vi "testArbNiTwoTone.vi"   [LabVIEW 2023]
uses:
  ArbNi.lvclass
  Data/arbWaveformType.ctl
  sweArb.lvlib
types:
  T1 = typedef "sweArb.lvlib/arbWaveformType.ctl" = enum16{"Sine", "Square", "Triangle", "DC", "Noise", "Arb"}
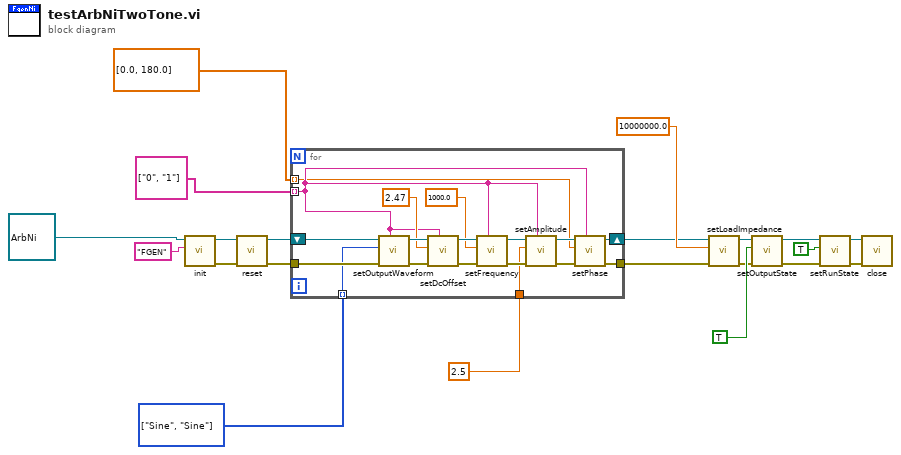
[diagram p0: block diagram]
diagram:
  w1 = T1[] [enum."Sine", enum."Sine"] items=["Sine", "Square", "Triangle", "DC", "Noise", "Arb"] ("Array")
  w9 = 10000000.0 items=["50 Ohm"=50.0, "High Z"=10000000.0] ("Load Impedance")
  n1 = call-dynamic "init.vi"("Resource"="FGEN", "FgenNiPxi in"=refnum<class "ArbNi.lvclass"> refnum) -> ("error out"=w20:errorcluster, "FgenNiPxi out"=w21:refnum<class "ArbNi.lvclass">)  [unwired: 8 in]
  n2 = call-dynamic "reset.vi"("error in (no error)"=w20, "FgenNiPxi in"=w21) -> ("error out"=w18:errorcluster, "FgenNiPxi out"=w19:refnum<class "ArbNi.lvclass">)  [unwired: 8 in]
  n3 = for {
    tunnel: w18 -> [w38]
    tunnel: [w30] -> w6
    tunnel: string[] ["0", "1"] ("Channel") -> [w26] mode=indexing
    tunnel: dbl[] [0.0, 180.0] ("Phase [°]") -> [w24] mode=indexing
    shift-right: [w31] -> w7
    shift-left: w19 -> [w39]
    tunnel: 2.5 ("Amplitude [Vpk]") -> [w23]
    tunnel: w1 -> [w22] mode=indexing
    n4 = call-dynamic "setOutputWaveform.vi"("Channel"=w26, "error in (no error)"=w38, "Type"=w22, "FgenNiPxi in"=w39) -> ("error out"=w36:errorcluster, "FgenNiPxi out"=w37:refnum<class "ArbNi.lvclass">)  [unwired: 6 in]
    n5 = call-dynamic "setDcOffset.vi"("Channel"=w26, "error in (no error)"=w36, "Offset [V]"=2.47, "FgenNiPxi in"=w37) -> ("error out"=w34:errorcluster, "FgenNiPxi out"=w35:refnum<class "ArbNi.lvclass">)  [unwired: 6 in]
    n6 = call-dynamic "setFrequency.vi"("Channel"=w26, "error in (no error)"=w34, "Frequency [Hz]"=1000.0, "FgenNiPxi in"=w35) -> ("error out"=w32:errorcluster, "FgenNiPxi out"=w33:refnum<class "ArbNi.lvclass">)  [unwired: 6 in]
    n7 = call-dynamic "setAmplitude.vi"("Channel"=w26, "error in (no error)"=w32, "Amplitude [Vpkpk]"=w23, "FgenNiPxi in"=w33) -> ("error out"=w25:errorcluster, "FgenNiPxi out"=w27:refnum<class "ArbNi.lvclass">)  [unwired: 6 in]
    n8 = call-dynamic "setPhase.vi"("Channel"=w26, "error in (no error)"=w25, "Phase [°]"=w24, "FgenNiPxi in"=w27) -> ("error out"=w30:errorcluster, "FgenNiPxi out"=w31:refnum<class "ArbNi.lvclass">)  [unwired: 6 in]
  }
  n9 = call-dynamic "setLoadImpedance.vi"("error in (no error)"=w6, "Load Impedance"=w9, "FgenNiPxi in"=w7) -> ("error out"=w5:errorcluster, "FgenNiPxi out"=w4:refnum<class "ArbNi.lvclass">)  [unwired: 7 in]
  n10 = call-dynamic "setOutputState.vi"("error in (no error)"=w5, "Output State"=TRUE, "FgenNiPxi in"=w4) -> ("error out"=w3:errorcluster, "FgenNiPxi out"=w17:refnum<class "ArbNi.lvclass">)  [unwired: 7 in]
  n11 = call-dynamic "setRunState.vi"("error in (no error)"=w3, "Runstate"=TRUE, "FgenNiPxi in"=w17) -> ("error out"=w11:errorcluster, "FgenNiPxi out"=w16:refnum<class "ArbNi.lvclass">)  [unwired: 7 in]
  n12 = call-dynamic "close.vi"("error in (no error)"=w11, "FgenNiPxi in"=w16) -> ()  [unwired: 9 in, 1 out]
